vi "sv_STFT by Indices.vi"(0 "scaled signal [EU]":waveform(dbl), 1 "indices":i32[](array[numeric]), 2 "FFT block size":i32=1024 min=1, 7 "weighting":T2 items=["Linear", "A-weighting", "B-weighting", "C-weighting", "ITU-R 468-4", "Dolby", "CCITT", "C-message"], 9 "window":T1=1 items=["Rectangle"=0, "Hanning"=1, "Hamming"=2, "Blackman-Harris"=3, "Exact Blackman"=4, "Blackman"=5, "Flat Top"=6, "4 Term B-Harris "=7, "7 Term B-Harris"=8, "Low Sidelobe"=9, "Blackman Nuttall"=11, "Triangle"=30, "Bartlett-Hanning"=31, "Bohman"=32, "Parzen"=33, "Welch"=34, "Kaiser"=60, "Dolph-Chebyshev"=61, "Gaussian"=62], 11 "error in (no error)":errorcluster, 12 "dB On (T)":bool=TRUE) -> (4 "power spectra [dB EU]":dbl[][](array[numeric]) format="%.2f", 6 "unit label":string, 8 "f0 and delta f [Hz]":cluster{"f0":dbl, "delta f":dbl} {"delta f" format="%.2f"; "f0" format="%.2f"}, 15 "error out":errorcluster)   [LabVIEW 2017]
uses:
  <vilib>/addons/Sound and Vibration/compatibility/Controls/svl_Weighting Filter Text Ring.ctl
  <vilib>/Analysis/4window.llb/windowTd.ctl
  <vilib>/addons/_NISVFA/_Baseband FFT/SVFA Power Spectrum (1 Ch).vi
  <vilib>/addons/Sound and Vibration/svt_Weighting/SoundVib_ABCWeighting.lvlib
  <vilib>/Analysis/NI_AALPro.lvlib
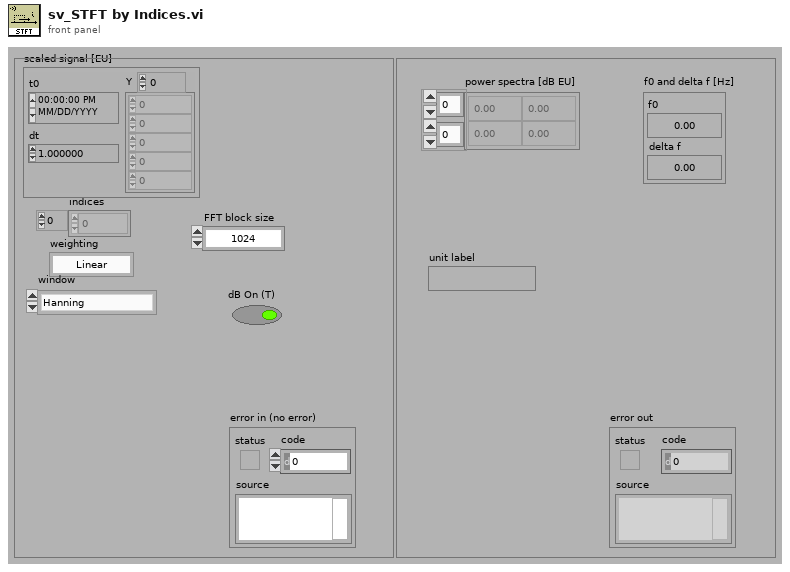
[diagram p1: front panel]
types:
  T1 = typedef "NI_AALPro.lvlib/windowTd.ctl" = u32
  T2 = typedef "svl_Weighting Filter Text Ring.ctl" = u16
  T3 = cluster{"averaging mode":enum16{"No averaging", "Vector averaging", "RMS averaging", "Peak hold"}, "weighting mode":enum16{"Linear", "Exponential"}, "number of averages":u32, "linear mode":enum16{"One shot", "Auto restart"}}
  T4 = typedef "svc_Spectrum Info.ctl" = cluster{"channel name":string, "description":string, "x-axis units":T5, "spectral info":cluster{"spectrum type":T6, "linear/dB":enum16{"linear", "dB"}, "window":u16, "window size":i32, "FFT size":i32}, "engineering units":T7, "custom label":string, "dB reference [EU]":dbl, "peak units":enum16{"rms", "peak", "peak-peak"}, "weighting filter":T8, "spectral density?":bool, "unit label":string, "spectrum skewed?":bool, "complimentary spectrum units":T9}
  T5 = typedef "svc_X-Axis Units.ctl" = u16
  T6 = typedef "svc_Spectrum Type.ctl" = enum16{"FFT Spectrum [complex]", "Amplitude [Magnitude]", "Power [Magnitude^2]", "Cross Spectrum [complex]", "Frequency Response [Complex]"}
  T7 = typedef "svc_Engineering Units Text Ring.ctl" = u16
  T8 = typedef "svc_Weighting Filter Text Ring.ctl" = u16
  T9 = typedef "svc_Complimentary Spectrum Units.ctl" = enum16{"none", "radians", "degrees", "cycles", "imaginary"}
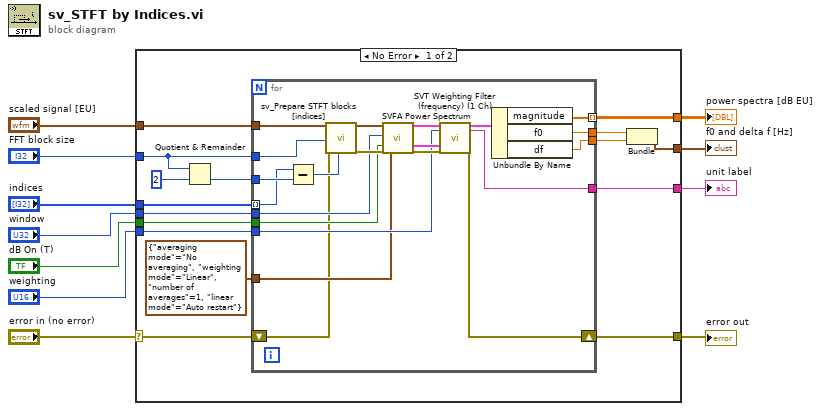
[diagram p0: block diagram]
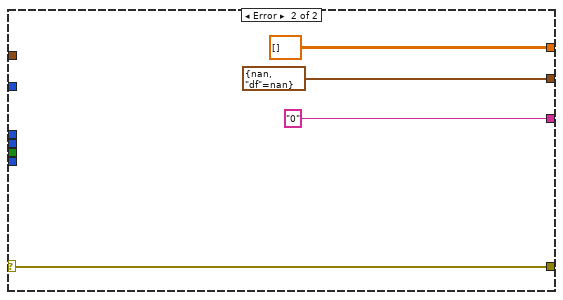
[diagram p2: hidden frame]
diagram:
  n1 = case shown="No Error" "error in (no error)" {
    selector: "error in (no error)" -> [w14 w49]
    tunnel: "FFT block size" -> [w25 _]
    tunnel: "dB On (T)" -> [w24 _]
    tunnel: "indices" -> [w23 _]
    tunnel: "scaled signal [EU]" -> [w22 _]
    tunnel: "window" -> [w21 _]
    tunnel: "weighting" -> [w20 _]
    tunnel: [w19 dbl[][] [] ("magnitude")] -> w5
    tunnel: [w18 "0" ("unit label")] -> w4
    tunnel: [w16 cluster{dbl, "df":dbl} {nan, "df"=nan}] -> w3
    tunnel: [w13 w49] -> w1
    frame No Error {
      n2 = Quotient & Remainder(x=w25, y=2) -> (floor(x/y)=w26:i32)  [unwired: 1 out]
      n3 = for {
        tunnel: w26 -> [w48]
        tunnel: w25 -> [w44]
        tunnel: w24 -> [w41]
        tunnel: w23 -> [w47] mode=indexing
        tunnel: w22 -> [w46]
        tunnel: w21 -> [w40]
        tunnel: w20 -> [w36]
        tunnel: [w35] -> w19 mode=indexing
        tunnel: [w34] -> w18
        tunnel: [w30] -> w17
        tunnel: T3 {"averaging mode"=enum."No averaging", "weighting mode"=enum."Linear", "number of averages"=1, "linear mode"=enum."Auto restart"} ("averaging parameters") -> [w33]
        shift-right: [w31] -> w13
        shift-left: w14 -> [w32]
        tunnel: [w28] -> w12
        n4 = Subtract(x=w47, y=w48) -> (x-y=w45:i32)
        n5 = call <vilib>:"sv_Prepare STFT blocks [indices].vi"("scaled signal [EU]"=w46, "FFT block size"=w44, "error in (no error)"=w32, "indices"=w45) -> ("scaled signal [EU]"=w43:waveform(dbl), "error out"=w42:errorcluster)  [unwired: 14 in]
        n6 = call-poly <vilib>:"SVFA Power Spectrum.vi"("scaled signal [EU]"=w43, "window"=w40, "dB On (T)"=w41, "error in (no error)"=w42, "averaging parameters"=w33) -> ("power spectrum [dB EU]"=w39:cluster{"f0":dbl, "df":dbl, "magnitude":dbl[]}, "spectrum info"=w38:T4, "error out"=w37:errorcluster)  [unwired: 9 in, 3 out]
        n7 = call <vilib>:"SVT Weighting Filter (frequency) (1 Ch).vi"("spectrum"=w39, "weighting"=w36, "spectrum info in"=w38, "error in (no error)"=w37) -> ("weighted spectrum"=w29:cluster{"f0":dbl, "df":dbl, "magnitude":dbl[]}, "unit label"=w34:string, "error out"=w31:errorcluster)  [unwired: 12 in, 1 out]
        n8 = Unbundle By Name(w29) -> ("magnitude"=w35:dbl[], "f0"=w28:dbl, "df"=w30:dbl)
      }
      n9 = Bundle("f0"=w12, "df"=w17) -> (w16:cluster{"f0":dbl, "df":dbl})  [unwired: 1 in]
    }
    frame Error {
    }
  }
  "power spectra [dB EU]" <- w5
  "f0 and delta f [Hz]" <- w3
  "unit label" <- w4
  "error out" <- w1
